vi "Encoder Example.vi"() -> ()   [LabVIEW 2012, in "Phidget Encoder.lvlib"]
uses:
  <instrlib>/Phidgets/Phidget Encoder/Phidget Encoder.lvlib
  <instrlib>/Phidgets/Phidget Encoder/Public/EncoderStart.vi
  <instrlib>/Phidgets/Phidget Encoder/Public/EncoderClose.vi
  <instrlib>/Phidgets/Phidget Common/Phidget Common.lvlib
panel:
  in  "stop":bool
  out "Position":i64
  out "error out":errorcluster
  in  "error in (no error)":errorcluster
  in  "Device Info":T1={"Serial Number"=-1, "Channel"=0, "Port"=0}
  out "Attached?":bool
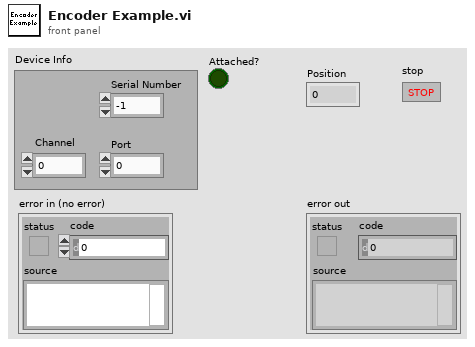
[diagram p1: front panel]
types:
  T1 = cluster{"Serial Number":i32, "Channel":i32, "Port":i32}
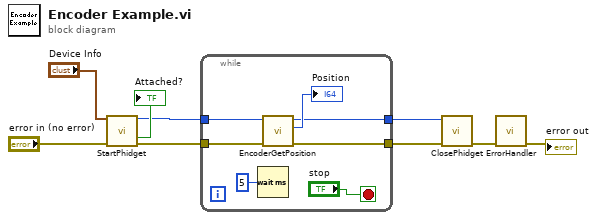
[diagram p0: block diagram]
diagram:
  n1 = call-poly <instrlib>:"StartPhidget.vi"("Device Info"="Device Info", "error in (no error)"="error in (no error)") -> ("Phidget ID"=w2:u64, "Attached?"=→"Attached?":bool, "error out"=w1:errorcluster)  [unwired: 10 in, 1 out]
  n2 = while {
    tunnel: [w11] -> w4
    tunnel: [w10] -> w3
    tunnel: w2 -> [w15]
    tunnel: w1 -> [w14]
    stop <- "stop" stop-if-true
    n3 = Wait (ms)(milliseconds to wait=u32 5) -> ()  [unwired: 1 out]
    n4 = call <instrlib>:"EncoderGetPosition.vi"("error in (no error)"=w14, "Device In"=w15) -> ("error out"=w10:errorcluster, "Position"=→"Position":i64, "Device Out"=w11:u64)  [unwired: 6 in]
  }
  n5 = call-poly <instrlib>:"ClosePhidget.vi"("error in"=w3, "Device In"=w4) -> ("error out"=w6:errorcluster)  [unwired: 9 in]
  n6 = call <instrlib>:"ErrorHandler.vi"("error in"=w6) -> ("error out"=→"error out":errorcluster)  [unwired: 9 in, 1 out]
